vi "ConnToMasterErr.vi"(11 "String":string) -> (3 "Abort?":bool)   [LabVIEW 2014]
doc: "Returns an error if there is no connection to the Master"
uses:
  <vilib>/Platform/browser.llb/Open URL in Default Browser (string).vi
panel:
  in  "OK Button":bool
  in  "Website":bool
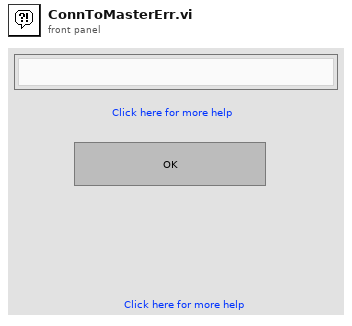
[diagram p1: front panel]
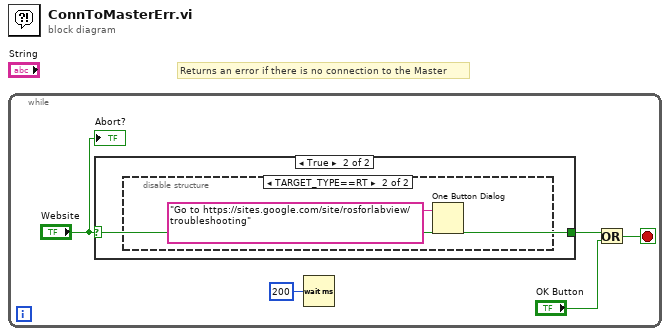
[diagram p0: block diagram]
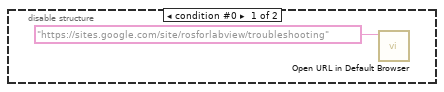
[diagram p3: hidden frame]
diagram:
  # "Returns an error if there is no connection to the Master"
  n1 = while {
    stop <- w2 stop-if-true
    n2 = case shown="True" "Website" {
      selector: "Website" -> [_ w6]
      tunnel: [_ w6] -> w3
      frame False {
      }
      frame True {
        n3 = disable-structure shown="TARGET_TYPE==RT" {
          frame condition #0 {
            n4 = call-poly <vilib>:"Open URL in Default Browser.vi"("URL"="https://sites.google.com/site/rosforlabview/troubleshooting") -> ()  [unwired: 5 in, 2 out]
          }
          frame condition #1 (active) {
            n5 = One Button Dialog(message="Go to https://sites.google.com/site/rosforlabview/troubleshooting") -> ()  [unwired: 1 in, 1 out]
          }
        }
      }
    }
    n6 = Wait (ms)(milliseconds to wait=u32 200) -> ()  [unwired: 1 out]
    n7 = Or(x=w3, y="OK Button") -> (x .or. y?=w2:bool)
    "Abort?" <- "Website"
  }
